vi "Build Scales.vi"(8 "error in":errorcluster, 11 "cfgFileIn":T1) -> (0 "error out":errorcluster, 2 "Scales":cluster{"trh":tag, "p":tag, "t":tag, "rh":tag}, 3 "cfgFileOut":T1)   [LabVIEW 2012, in "CRDS.lvclass"]
doc: "Using the config file, build the scales as necessary. There are currently 4 scales that are used to scale measurements off of the housekeeping cards. The scales are for the temperature on the Vaisala probe, the RH on the Vaisala probe, pressure from the Honeywell pressure transducers and the temperature from the thermistors. Each scale is applied to the actual measurement such that the value that is retrieved from the card is the actual scaled value rather than the voltage. \nIn order to retrieve the voltage from the card, apply the scale in an inverted manner."
uses:
  CRDS.lvclass
  <vilib>/DAQmx/create/scale.llb/DAQmx Create Scale (Linear).vi
  General/Temperature/Temperature.lvlib
  General/Temperature/Thermistor Config.ctl
  PAS/Controls/Configuration/Thermistor.ctl
  General/Atmospheric/Atmospheric Constants.vi
  General/Atmospheric/Atmospheric Library.lvlib
  <vilib>/DAQmx/create/scale.llb/DAQmx Create Scale (Table).vi
  <vilib>/Utility/config.llb/Config Data RefNum.ctl
  <vilib>/Utility/config.llb/NI_LVConfig.lvlib
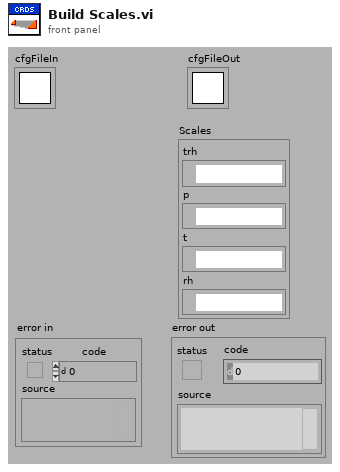
[diagram p1: front panel]
types:
  T1 = typedef "NI_LVConfig.lvlib/Config Data RefNum.ctl" = refnum<k1>
  T2 = typedef "Thermistor.ctl" = cluster{"R1":sgl, "Vs":sgl, "Rref":sgl[], "Tref":sgl[]}
  T3 = typedef "Temperature.lvlib/Thermistor Config.ctl" = cluster{"Vsource":dbl, "SH Coeff":dbl[], "R1":dbl, "Rref":dbl[], "Tref":dbl[]}
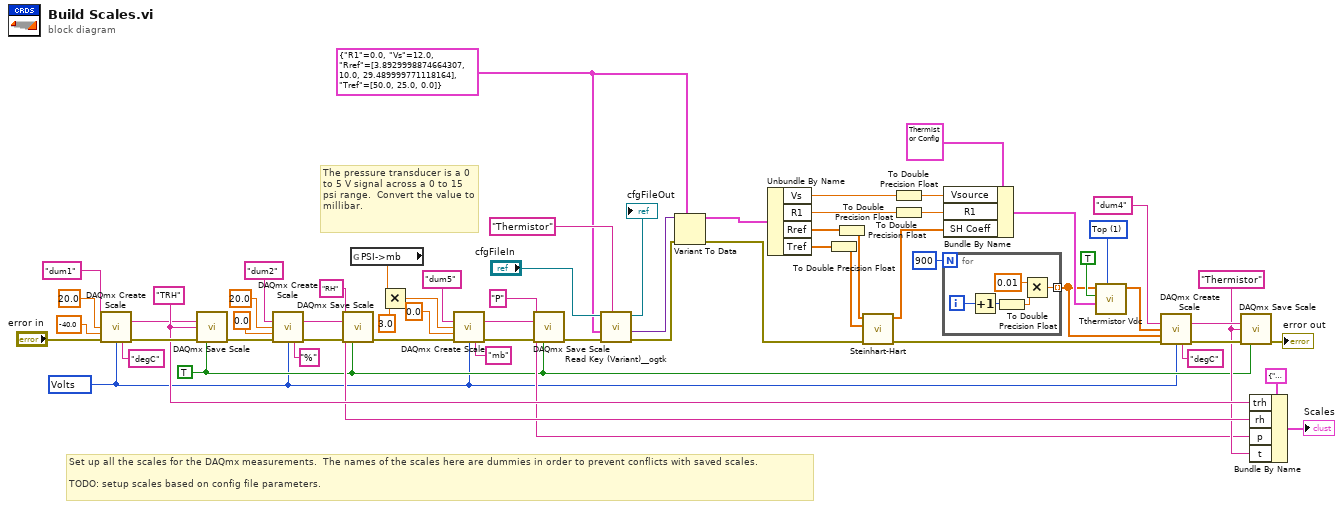
[diagram p0: block diagram]
diagram:
  w16 = u16 1 items=["Bottom", "Top"] ("ThermConfig")
  w30 = "P" ("name")
  w1 = T2 {"R1"=0.0, "Vs"=12.0, "Rref"=[3.893, 10.0, 29.49], "Tref"=[50.0, 25.0, 0.0]} ("Thermistor")
  w39 = "Thermistor" ("name")
  w41 = "RH" ("name")
  w43 = "TRH" ("name")
  w19 = TRUE ("overwrite existing scale?")
  w18 = 10348 items=["Volts"=10348, "Amps"=10342, "Deg F"=10144, "Deg C"=10143, "Deg R"=10145, "Kelvins"=10325, "Strain"=10299, "Ohms"=10384, "Hz"=10373, "Seconds"=10364, "Meters"=10219, "Inches"=10379, "Degrees"=10146, "Radians"=10273, "g"=10186, "m/s^2"=12470, "Pascals"=10081, "From TEDS"=12516] ("pre-scaled units")
  # "The pressure transducer is a 0 to 5 V signal across a 0 to 15 psi range.  Convert the value to millibar."
  # "Set up all the scales for the DAQmx measurements.  The names of the scales here are dummies in order to prevent conflicts with saved scales.\n\nTODO: setup scales based on config file parameters."
  n1 = call-poly <vilib>:"DAQmx Create Scale.vi"("name"="dum1", "slope"=20.0, "y-intercept"=-40.0, "error in"="error in", "pre-scaled units"=w18, "scaled units"="degC") -> ("scale out"=w29:tag, "error out"=w47:errorcluster)  [unwired: 8 in]
  n2 = call <vilib>:"DAQmx Save Scale.vi"("scale name"=w29, "save as"=w43, "error in"=w47, "overwrite existing scale?"=w19) -> ("error out"=w27:errorcluster)  [unwired: 11 in]
  n3 = call-poly <vilib>:"DAQmx Create Scale.vi"("name"="dum2", "slope"=20.0, "y-intercept"=0.0, "error in"=w27, "pre-scaled units"=w18, "scaled units"="%") -> ("scale out"=w49:tag, "error out"=w46:errorcluster)  [unwired: 8 in]
  n4 = call <vilib>:"DAQmx Save Scale.vi"("scale name"=w49, "save as"=w41, "error in"=w46, "overwrite existing scale?"=w19) -> ("error out"=w26:errorcluster)  [unwired: 11 in]
  n5 = global read "Atmospheric Constants.vi" "PSI->mb"() -> (w3:sgl)
  n6 = Multiply(x=w3, y=3.0 ("slope")) -> (x*y=w31:dbl)
  n7 = call-poly <vilib>:"DAQmx Create Scale.vi"("name"="dum5", "slope"=w31, "y-intercept"=0.0, "error in"=w26, "pre-scaled units"=w18, "scaled units"="mb") -> ("scale out"=w34:tag, "error out"=w35:errorcluster)  [unwired: 8 in]
  n8 = call <vilib>:"DAQmx Save Scale.vi"("scale name"=w34, "save as"=w30, "error in"=w35, "overwrite existing scale?"=w19) -> ("error out"=w7:errorcluster)  [unwired: 11 in]
  n9 = call <userlib>:"Read Key (Variant)__ogtk.vi"("section"="Thermistor", "error in (no error)"=w7, "type"=w1, "refnum"="cfgFileIn") -> ("error out"=w6:errorcluster, "key-value"=w20:variant, "refnum out"=→"cfgFileOut":T1)  [unwired: 4 in, 1 out]
  n10 = Variant To Data(error in=w6, type=w1, Variant=w20) -> (data=w23:T2, error out=w5:errorcluster)
  n11 = Unbundle By Name(w23) -> ("Vs"=w14:sgl, "R1"=w13:sgl, "Rref"=w11:sgl[], "Tref"=w9:sgl[])
  n12 = To Double Precision Float(number=w9) -> (double precision float=w8:dbl[])
  n13 = To Double Precision Float(number=w11) -> (double precision float=w10:dbl[])
  n14 = call "Steinhart-Hart.vi"("error in"=w5, "Tref (C)"=w8, "R (kO)"=w10) -> ("error out"=w28:errorcluster, "Coefficients"=w53:dbl[])  [unwired: 7 out]
  n15 = To Double Precision Float(number=w14) -> (double precision float=w15:dbl)
  n16 = To Double Precision Float(number=w13) -> (double precision float=w12:dbl)
  n17 = for {
    N: 900 -> [_]
    tunnel: [w66] -> w51 mode=indexing
    i -> [w65]
    n18 = Increment(x=w65) -> (x+1=w64:i32)
    n19 = To Double Precision Float(number=w64) -> (double precision float=w63:dbl)
    n20 = Multiply(x=0.01, y=w63) -> (x*y=w66:dbl)
  }
  n21 = Bundle By Name(cluster=T3 {"Vsource"=12.0, "SH Coeff"=[2.7200000286102295], "R1"=10.0, "Rref"=[], "Tref"=[]} ("Thermistor Circuit"), "Vsource"=w15, "R1"=w12, "SH Coeff"=w53) -> (w55:T3)
  n22 = call "Tthermistor Vdc.vi"("ThermConfig"=w16, "thermCirc"=w55, "Init"=TRUE ("Initialize"), "Vdc"=w51) -> ("T"=w50:dbl[])  [unwired: 4 in, 1 out]
  n23 = call-poly <vilib>:"DAQmx Create Scale.vi"("name"="dum4", "scaled values"=w50, "pre-scaled values"=w51, "error in"=w28, "pre-scaled units"=w18, "scaled units"="degC") -> ("scale out"=w48:tag, "error out"=w45:errorcluster)  [unwired: 8 in]
  n24 = call <vilib>:"DAQmx Save Scale.vi"("scale name"=w48, "save as"=w39, "error in"=w45, "overwrite existing scale?"=w19) -> ("error out"=→"error out":errorcluster)  [unwired: 11 in]
  n25 = Bundle By Name(cluster=cluster{"trh":tag, "p":tag, "t":tag, "rh":tag} {"trh"="", "p"="", "t"="", "rh"=""} ("input cluster"), "trh"=w43, "rh"=w41, "p"=w30, "t"=w39) -> (→"Scales":cluster{"trh":tag, "p":tag, "t":tag, "rh":tag})
